vi "Launch.vi"   [LabVIEW 2020, in "Application.lvclass"]
uses:
  Application.lvclass
  Container/View/View.lvclass
panel:
  # "LAUNCHER"
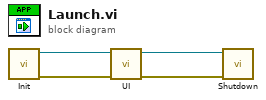
[diagram p0: block diagram]
diagram:
  n1 = call "Init.vi"() -> ("error out"=w3:errorcluster, "View out"=w4:refnum<class "View.lvclass">)  [unwired: 10 in]
  n2 = call "UI.vi"("error in (no error)"=w3, "View in"=w4) -> ("error out"=w1:errorcluster, "View out"=w2:refnum<class "View.lvclass">)  [unwired: 8 in]
  n3 = call "Shutdown.vi"("error in (no error)"=w1, "View in"=w2) -> ()  [unwired: 8 in, 2 out]
